vi "WriteTxt.vi"() -> ()   [LabVIEW 2014]
panel:
  in  "Path":path
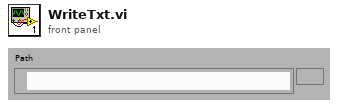
[diagram p1: front panel]
types:
  T1 = enum16{"open", "replace", "create", "open or create", "replace or create", "replace or create with confirmation"}
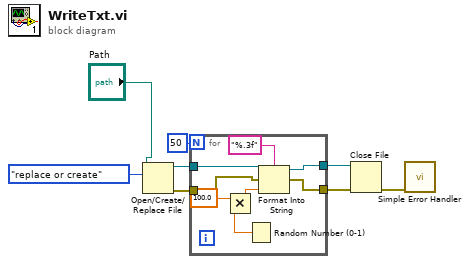
[diagram p0: block diagram]
diagram:
  n1 = Open/Create/Replace File(file path (use dialog)="Path", operation (0:open)=T1."replace or create") -> (refnum out=w7:refnum<file>, error out=w6:errorcluster)  [unwired: 4 in, 1 out]
  n2 = for {
    N: 50 -> [_]
    tunnel: w7 -> [w16]
    tunnel: w6 -> [w13]
    tunnel: [w15] -> w4
    tunnel: [w14] -> w5
    n3 = Random Number (0-1)() -> (number: 0 to 1=w12:dbl)
    n4 = Multiply(x=100.0, y=w12) -> (x*y=w10:dbl)
    n5 = Format Into String(format string="%.3f", initial string=w16, error in=w13, w10) -> (resulting string=w15:refnum<file>, error out=w14:errorcluster)
  }
  n6 = Close File(refnum=w4, error in=w5) -> (error out=w3:errorcluster)  [unwired: 1 out]
  n7 = call <vilib>:"Simple Error Handler.vi"("error in (no error)"=w3) -> ()  [unwired: 4 in, 5 out]
